vi "AMG88338x8ThermalCamera.vi"() -> ()   [LabVIEW 2024]
uses:
  Driver/Public/Digital Pull Direction.ctl
  1e6ec9c9-fb05-4fd0-b05f-9caec19ae962.vi
  <vilib>/gmath/interp.llb/Interpolate 2D (2d X,Y).vi
  <vilib>/gmath/NI_Gmath.lvlib
  Driver/CTIPicoVISA.lvlib
panel:
  out "error out":errorcluster
  in  "Colormap Name":T1(ring)=enum."vanimo"
  out "Intensity Graph 2":dbl[][](graph)
  in  "Grove Connector":enum16{"I2C0", "I2C1"}(ring)
  in  "VISA resource name in":refnum<visa-resource-name>="COM10"
  out "Thermistor Value":dbl
  in  "method":i32(ring)=3 items=["nearest", "bilinear", "bicubic", "bicubic spline"]
  out "LoopIndex":i32
  in  "Stop":bool
  out "Intensity Graph":dbl[][](graph)
  out "Identity":T2
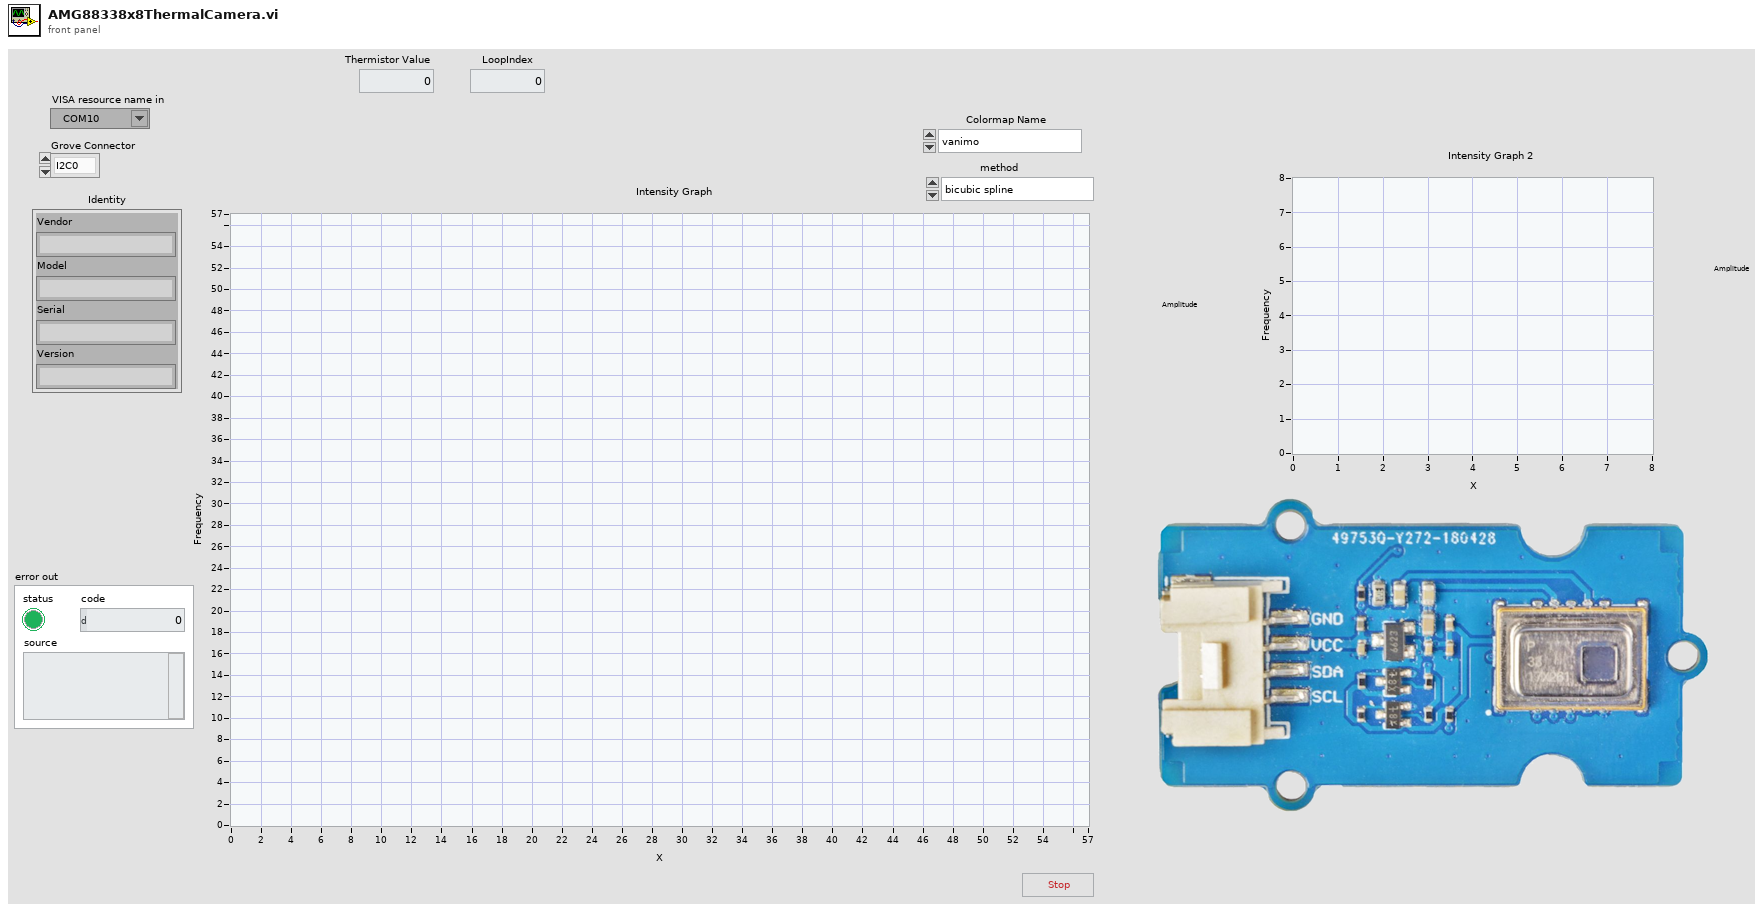
[diagram p1: front panel]
types:
  T1 = enum16{"magma", "inferno", "plasma", "viridis", "cividis", "twilight", "twilight_shifted", "turbo", "berlin", "managua", "vanimo"}
  T2 = cluster{"Vendor":string, "Model":string, "Serial":string, "Version":string}
  T3 = typedef "CTIPicoVISA.lvlib/Digital Pull Direction.ctl" = enum16{"None", "Up", "Down", "Both"}
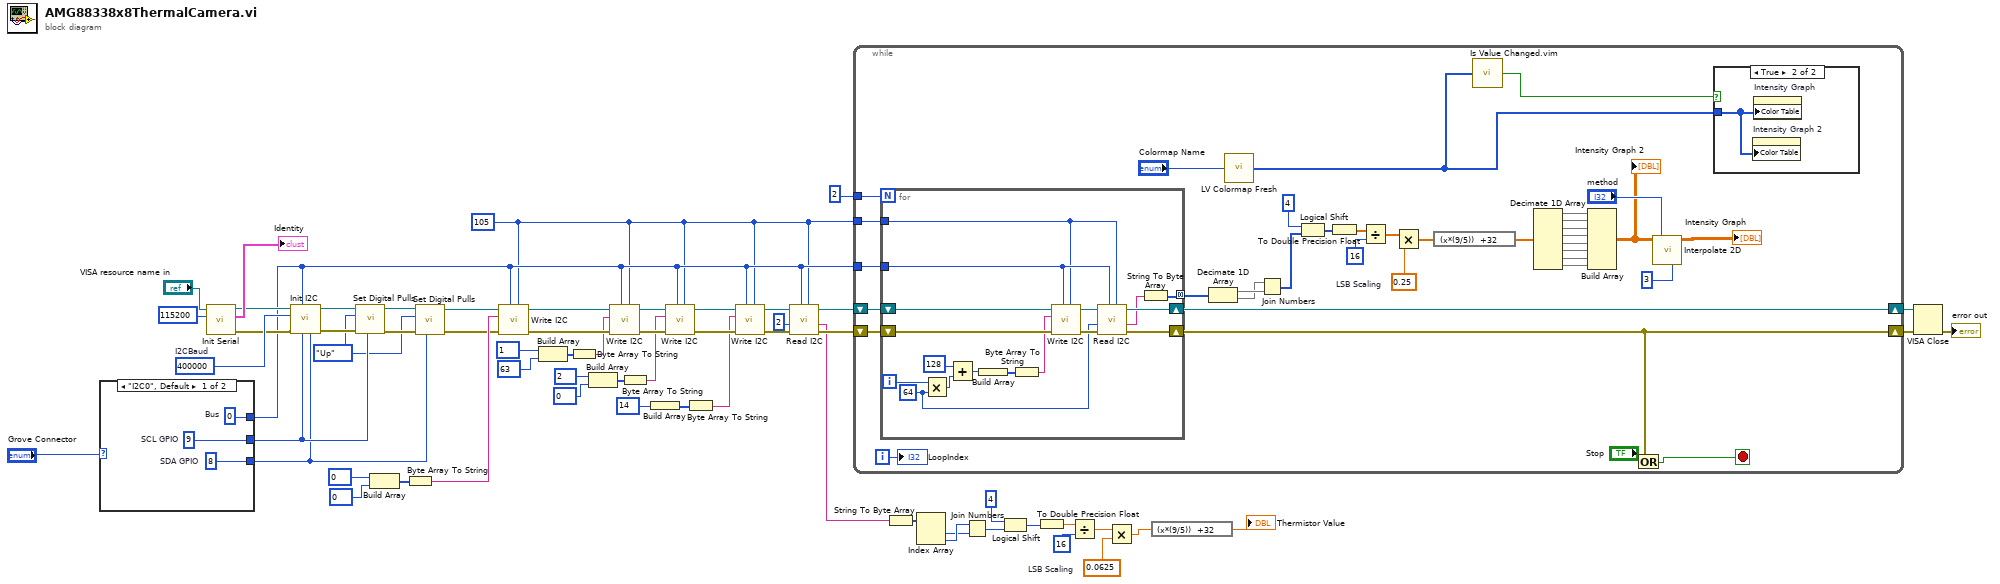
[diagram p0: block diagram]
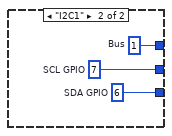
[diagram p2: hidden frame]
diagram:
  w16 = Digital_Pull_Direction."Up" ("Pull")
  w23 = u32 400000  # I2CBaud
  w26 = 0.0625  # LSB Scaling
  w3 = u8 105 ("Address")
  n1 = case shown="\"I2C0\", Default" "Grove Connector" {
    tunnel: [w64 w67] -> w17
    tunnel: [w63 w66] -> w15
    tunnel: [w62 w65] -> w4
    frame "I2C0", Default {
      w62 = u8 0  # Bus
      w63 = 8  # SDA GPIO
      w64 = 9  # SCL GPIO
    }
    frame "I2C1" {
      w65 = u8 1  # Bus
      w66 = 6  # SDA GPIO
      w67 = 7  # SCL GPIO
    }
  }
  n2 = call "Init Serial.vi"("Baud (115200)"=u32 115200, "VISA resource name in"="VISA resource name in") -> ("error out"=w10:errorcluster, "Identity"=→"Identity":T2, "VISA resource name Out"=w11:refnum<visa-resource-name>)  [unwired: 7 in]
  n3 = call "Init I2C.vi"("SDA GPIO"=w15, "SCL GPIO"=w17, "Bus"=w4, "error in (no error)"=w10, "Baud"=w23, "VISA resource name in"=w11) -> ("error out"=w20:errorcluster, "VISA resource name"=w21:refnum<visa-resource-name>)  [unwired: 4 in]
  n4 = call "Set Digital Pulls.vi"("GPIO"=w17, "error in (no error)"=w20, "Pull"=w16, "VISA resource name in"=w21) -> ("error out"=w18:errorcluster, "VISA resource name"=w19:refnum<visa-resource-name>)  [unwired: 6 in]
  n5 = Build Array(u8 0 ("Address"), u8 0 ("Address")) -> (w58:u8[])
  n6 = Byte Array To String(unsigned byte array=w58) -> (string=w61:string)
  n7 = call "Set Digital Pulls.vi"("GPIO"=w15, "error in (no error)"=w18, "Pull"=w16, "VISA resource name in"=w19) -> ("error out"=w12:errorcluster, "VISA resource name"=w13:refnum<visa-resource-name>)  [unwired: 6 in]
  n8 = call "Write I2C.vi"("Address"=w3, "Bus"=w4, "error in (no error)"=w12, "Data"=w61, "VISA resource name in"=w13) -> ("error out"=w57:errorcluster, "VISA resource name"=w52:refnum<visa-resource-name>)  [unwired: 5 in]
  n9 = Build Array(u8 1 ("Address"), u8 63 ("Address")) -> (w51:u8[])
  n10 = Byte Array To String(unsigned byte array=w51) -> (string=w48:string)
  n11 = Build Array(u8 2 ("Address"), u8 0 ("Address")) -> (w43:u8[])
  n12 = call "Write I2C.vi"("Address"=w3, "Bus"=w4, "error in (no error)"=w57, "Data"=w48, "VISA resource name in"=w52) -> ("error out"=w53:errorcluster, "VISA resource name"=w46:refnum<visa-resource-name>)  [unwired: 5 in]
  n13 = Byte Array To String(unsigned byte array=w43) -> (string=w42:string)
  n14 = Build Array(u8 14 ("Address")) -> (w39:u8[])
  n15 = call "Write I2C.vi"("Address"=w3, "Bus"=w4, "error in (no error)"=w53, "Data"=w42, "VISA resource name in"=w46) -> ("error out"=w47:errorcluster, "VISA resource name"=w41:refnum<visa-resource-name>)  [unwired: 5 in]
  n16 = Byte Array To String(unsigned byte array=w39) -> (string=w38:string)
  n17 = call "Write I2C.vi"("Address"=w3, "Bus"=w4, "error in (no error)"=w47, "Data"=w38, "VISA resource name in"=w41) -> ("error out"=w6:errorcluster, "VISA resource name"=w7:refnum<visa-resource-name>)  [unwired: 5 in]
  n18 = call "Read I2C.vi"("Address"=w3, "Bus"=w4, "error in (no error)"=w6, "Len"=u8 2 ("Read Len"), "VISA resource name in"=w7) -> ("error out"=w9:errorcluster, "Data"=w2:string, "VISA resource name"=w8:refnum<visa-resource-name>)  [unwired: 4 in]
  n19 = while {
    tunnel: 2 -> [w104]
    tunnel: w4 -> [w89]
    tunnel: w3 -> [w88]
    shift-right: [w84] -> w55
    shift-left: w9 -> [w91]
    shift-right: [w92] -> w54
    shift-left: w8 -> [w90]
    i -> [w86]
    stop <- w85 stop-if-true
    w72 = 0.25  # LSB Scaling
    n20 = for {
      N: w104 -> [_]
      shift-right: [w109] -> w84
      shift-left: w91 -> [w119]
      shift-right: [w111] -> w92
      shift-left: w90 -> [w120]
      tunnel: w89 -> [w108]
      tunnel: w88 -> [w107]
      tunnel: [w121] -> w103 mode=concatenating
      i -> [w116]
      w106 = u8 64 ("Read Len")
      n21 = Multiply(x=w116, y=w106) -> (x*y=w114:i32)
      n22 = Add(x=u8 128 ("Address"), y=w114) -> (x+y=w115:i32)
      n23 = Build Array(w115) -> (w122:i32[])
      n24 = Byte Array To String(unsigned byte array=w122) -> (string=w118:string)
      n25 = call "Write I2C.vi"("Address"=w107, "Bus"=w108, "error in (no error)"=w119, "Data"=w118, "VISA resource name in"=w120) -> ("error out"=w113:errorcluster, "VISA resource name"=w112:refnum<visa-resource-name>)  [unwired: 5 in]
      n26 = call "Read I2C.vi"("Address"=w107, "Bus"=w108, "error in (no error)"=w113, "Len"=w106, "VISA resource name in"=w112) -> ("error out"=w109:errorcluster, "Data"=w110:string, "VISA resource name"=w111:refnum<visa-resource-name>)  [unwired: 4 in]
      n27 = String To Byte Array(string=w110) -> (unsigned byte array=w121:u8[])
    }
    n28 = Decimate 1D Array(w103) -> (w102:u8[], w101:u8[])
    n29 = call "LV Colormap Fresh.vi"("Colormap Name"="Colormap Name") -> ("Colormap"=w68:u32[])  [unwired: 14 in]
    n30 = Join Numbers(hi=w101, lo=w102) -> ((hi.lo)=w79:u16[])
    n31 = Logical Shift(y=i16 4, x=w79) -> (x << y=w82:u16[])
    n32 = To Double Precision Float(number=w82) -> (double precision float=w81:dbl[])
    n33 = Divide(x=w81, y=i16 16) -> (x/y=w78:dbl[])
    n34 = Multiply(x=w78, y=w72) -> (x*y=w73:dbl[])
    n35 = expression code="(x*(9/5))  +32"(w73) -> (w77:dbl[])
    n36 = call "Is Value Changed.vim"("value"=w68) -> ("changed or first call?"=w74:bool)
    n37 = Decimate 1D Array(w77) -> (w93:dbl[], w94:dbl[], w95:dbl[], w96:dbl[], w97:dbl[], w98:dbl[], w99:dbl[], w100:dbl[])
    n38 = Build Array(w93, w94, w95, w96, w97, w98, w99, w100) -> (w70:dbl[][])
    "Intensity Graph 2" <- w70
    n39 = Or(x="Stop", y=w84) -> (x .or. y?=w85:bool)
    n40 = call-poly <vilib>:"Interpolate 2D.vi"("ntimes"=3, "method"="method", "Z"=w70) -> ("zi"=→"Intensity Graph":dbl[][])  [unwired: 5 in, 3 out]
    n41 = case shown="True" w74 {
      tunnel: w68 -> [_ w105]
      frame False {
      }
      frame True {
        n42 = property on="Intensity Graph 2" class="IntGraph (strict)"("Color Table"=w105) -> ()  [unwired: 2 in, 2 out]
        n43 = property on="Intensity Graph" class="IntGraph (strict)"("Color Table"=w105) -> ()  [unwired: 2 in, 2 out]
      }
    }
    "LoopIndex" <- w86
  }
  n44 = String To Byte Array(string=w2) -> (unsigned byte array=w37:u8[])
  n45 = Index Array(array=w37) -> (element #1=w35:u8, element #2=w36:u8)  [unwired: 2 in]
  n46 = Join Numbers(hi=w36, lo=w35) -> ((hi.lo)=w28:u16)
  n47 = Logical Shift(y=i16 4, x=w28) -> (x << y=w31:u16)
  n48 = To Double Precision Float(number=w31) -> (double precision float=w32:dbl)
  n49 = Divide(x=w32, y=i16 16) -> (x/y=w34:dbl)
  n50 = Multiply(x=w34, y=w26) -> (x*y=w27:dbl)
  n51 = expression code="(x*(9/5))  +32"(w27) -> (→"Thermistor Value":dbl)
  n52 = VISA Close(VISA resource name=w54, error in (no error)=w55) -> (error out=→"error out":errorcluster)
